vi "Smooth Ramp by Samples.vi"(8 "error in (no error)":errorcluster, 9 "End":dbl[](array[numeric]), 10 "Start":dbl[](array[numeric]), 11 "Instrument.DAQ":refnum<class "Instrument.DAQ.lvclass">) -> (0 "Error out":errorcluster, 2 "Waveforms out":waveform(dbl)[](array[waveform]), 3 "Instrument.DAQ out":refnum<class "Instrument.DAQ.lvclass">)   [LabVIEW 2019, in "Instrument.Lockin.lvlib" / "Instrument.DAQ.lvclass"]
uses:
  Instrument.DAQ.lvclass
  Instrument.DAQ.lvclass/Instrument.DAQ.ctl
  <vilib>/Analysis/NI_AALBase.lvlib
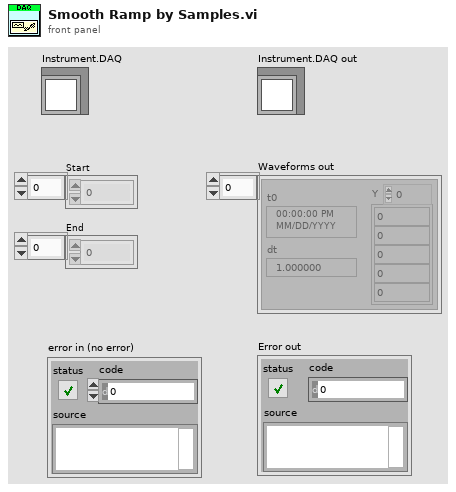
[diagram p1: front panel]
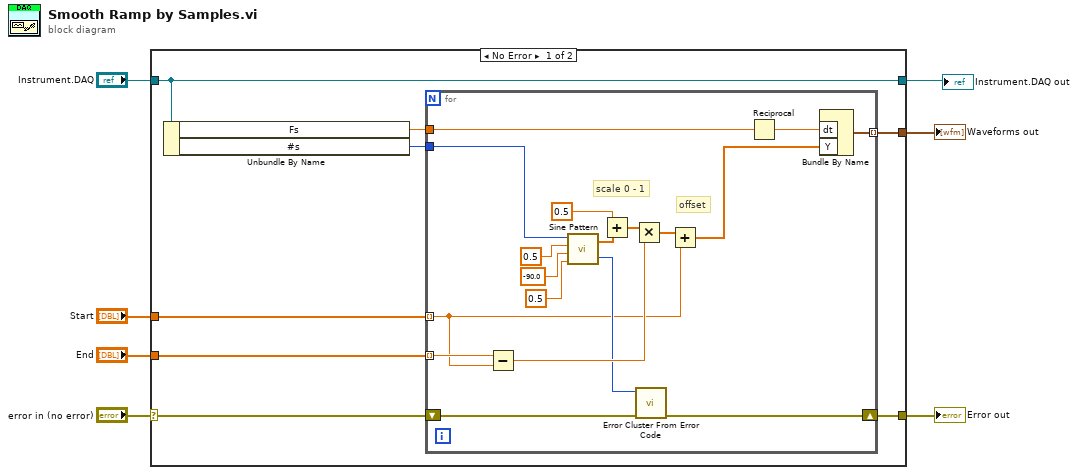
[diagram p0: block diagram]
diagram:
  n1 = case shown="No Error" "error in (no error)" {
    selector: "error in (no error)" -> [w13 w35]
    tunnel: "End" -> [w15 _]
    tunnel: [w14 w35] -> w5
    tunnel: [w11 _] -> w4
    tunnel: "Instrument.DAQ" -> [w9 w34]
    tunnel: [w9 w34] -> w2
    tunnel: "Start" -> [w8 _]
    frame No Error {
      n2 = Unbundle By Name(w9) -> ("Fs"=w12:dbl, "#s"=w10:i32)
      n3 = for {
        tunnel: w15 -> [w25] mode=indexing
        tunnel: w12 -> [w19]
        tunnel: [w18] -> w11 mode=indexing
        tunnel: w10 -> [w17]
        shift-right: [w23] -> w14
        shift-left: w13 -> [w22]
        tunnel: w8 -> [w16] mode=indexing
        # "offset"
        # "scale 0 - 1"
        n4 = Subtract(x=w25, y=w16) -> (x-y=w31:dbl)
        n5 = call <vilib>:"Sine Pattern.vi"("cycles"=0.5 ("cycles 2"), "phase(degrees)"=-90.0, "amplitude"=0.5, "samples"=w17) -> ("error"=w24:i32, "Sinusoidal Pattern"=w27:dbl[])
        n6 = Add(x=0.5 ("cycles 2"), y=w27) -> (x+y=w30:dbl[])
        n7 = Multiply(x=w30, y=w31) -> (x*y=w32:dbl[])
        n8 = call <vilib>:"Error Cluster From Error Code.vi"("error in (no error)"=w22, "error code (0)"=w24) -> ("error out"=w23:errorcluster)  [unwired: 7 in]
        n9 = Add(x=w32, y=w16) -> (x+y=w20:dbl[])
        n10 = Reciprocal(x=w19) -> (1/x=w21:dbl)
        n11 = Bundle By Name("dt"=w21, "Y"=w20) -> (w18:waveform(dbl))  [unwired: 1 in]
      }
    }
    frame Error {
    }
  }
  "Waveforms out" <- w4
  "Error out" <- w5
  "Instrument.DAQ out" <- w2
